vi "Check RPM.vi"(10 "RPM Wanted":dbl, 11 "Execute?":bool) -> (3 "Done":bool)   [LabVIEW 2012]
uses:
  Globals/Useful Values.vi
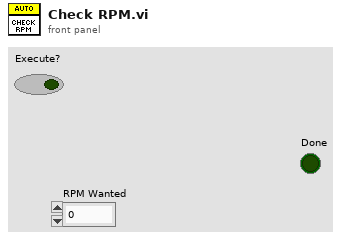
[diagram p1: front panel]
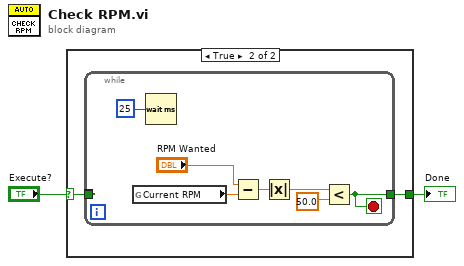
[diagram p0: block diagram]
diagram:
  n1 = case shown="True" "Execute?" {
    selector: "Execute?" -> [w3 w4]
    tunnel: [w3 w5] -> w1
    frame False {
    }
    frame True {
      n2 = while {
        tunnel: [w7] -> w5
        tunnel: [w6] -> _
        tunnel: w4 -> [w6]
        stop <- w7 stop-if-true
        n3 = global read "Useful Values.vi" "Current RPM"() -> (w11:dbl)
        n4 = Wait (ms)(milliseconds to wait=u32 25) -> ()  [unwired: 1 out]
        n5 = Subtract(x="RPM Wanted", y=w11) -> (x-y=w10:dbl)
        n6 = Absolute Value(x=w10) -> (abs(x)=w9:dbl)
        n7 = Less?(x=w9, y=50.0) -> (x < y?=w7:bool)
      }
    }
  }
  "Done" <- w1
